vi "SerialServer.vi"(4 "STOP REF":refnum<vi>, 6 "Local Port":u16=16505, 7 "FPGA REF (DBDE)":T1) -> ()   [LabVIEW 2015]
uses:
  Controls (HOST)/FPGA REF (MWT).ctl
panel:
  out "Baud Rate":i32(ring)=1 items=["9600"=1, "19200"=2, "38400"=4, "57600"=8, "115200"=16, "230400"=32, "460800"=64, "921600"=128]
  out "error out":errorcluster
  out "OverRunError":bool
  in  "Flush on Close":bool
  out "UART TX count":u64
  out "UART RX count":u64
  out "TCP Bytes Out":u64
  out "Elements in UART TX Queue":i32
  out "Elements in UART RX Queue":i32
  out "TCP Bytes In":u64
  out "connection ID":refnum<k5>
  out "Connected?":bool
  out "Stopped?":bool caption="BeenStopped?"
  out "Remote Address":string
  out "Remote Port":u16
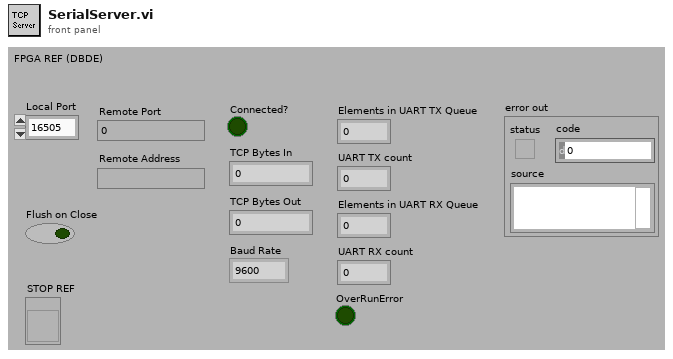
[diagram p1: front panel]
types:
  T1 = typedef "FPGA REF (MWT).ctl" = refnum<k20>
  T2 = enum16{"Standard", "Buffered", "CRLF", "Immediate"}
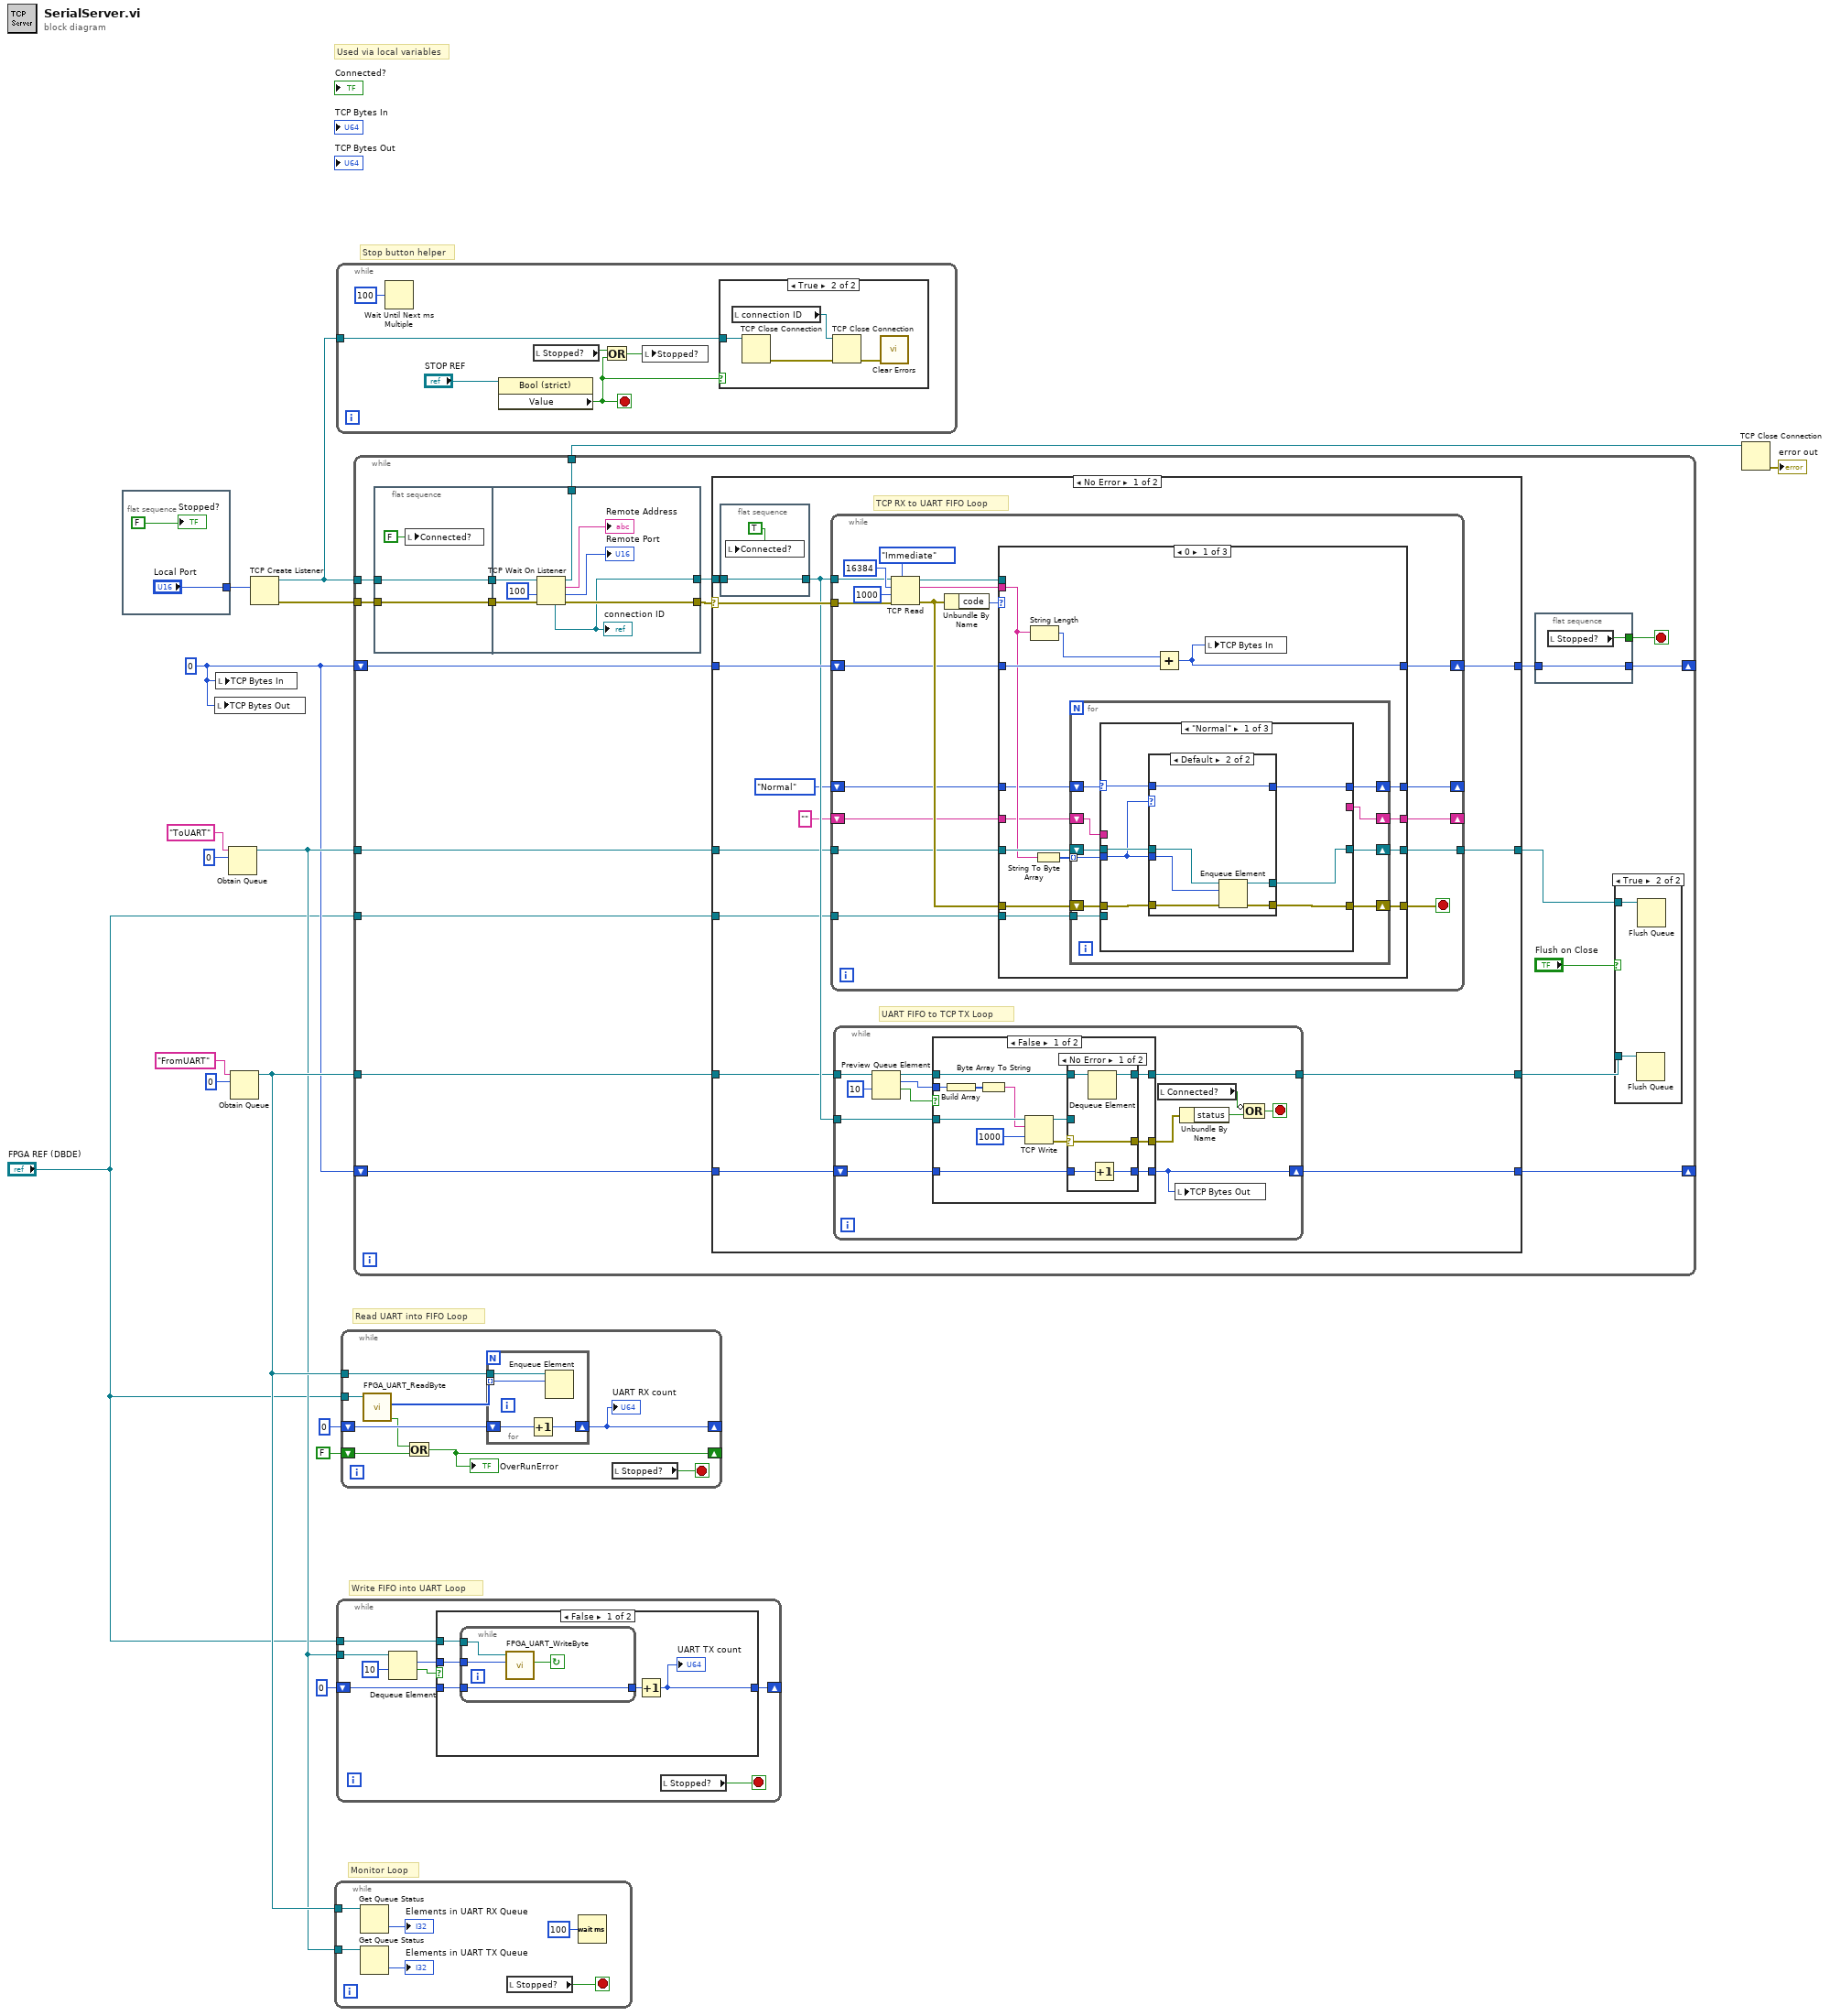
[diagram p0: block diagram]
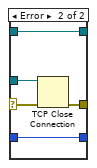
[diagram p5: hidden frame]
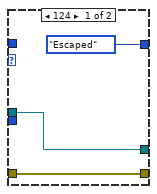
[diagram p7: hidden frame]
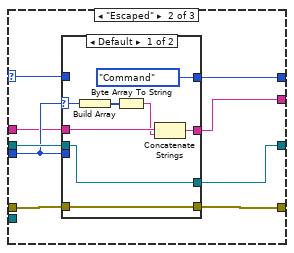
[diagram p8: hidden frame]
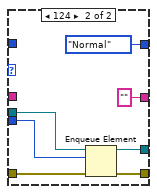
[diagram p9: hidden frame]
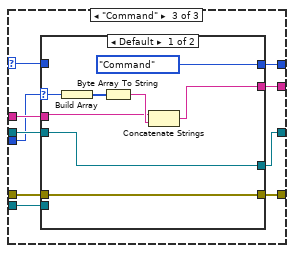
[diagram p10: hidden frame]
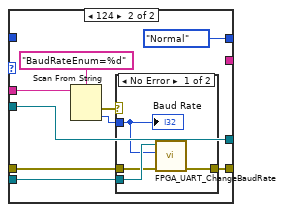
[diagram p11: hidden frame]
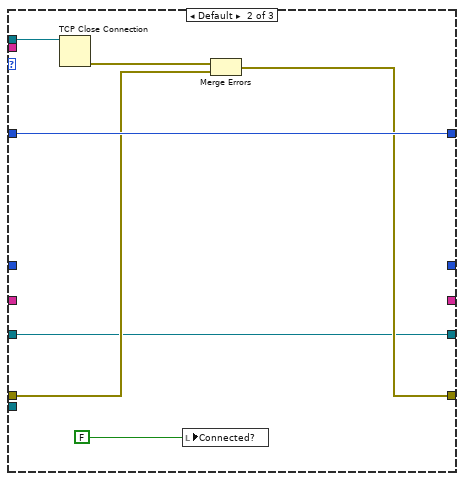
[diagram p13: hidden frame]
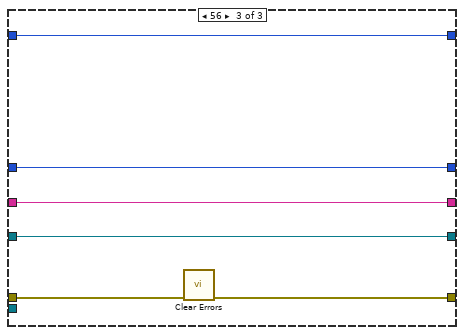
[diagram p14: hidden frame]
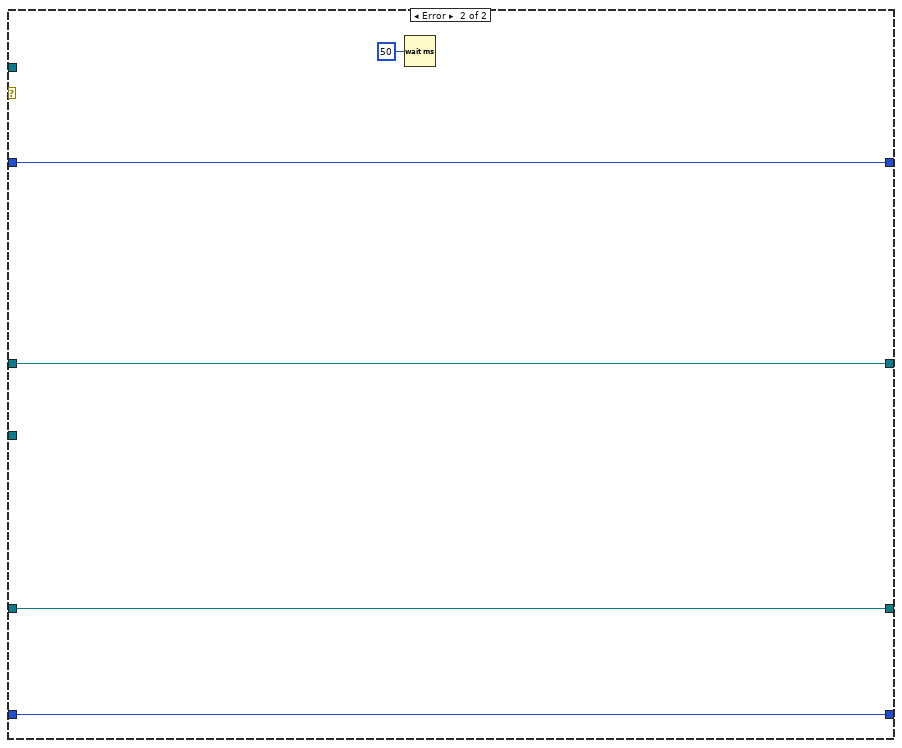
[diagram p15: hidden frame]
diagram:
  w8 = u64 0
  # "Monitor Loop"
  # "Write FIFO into UART Loop"
  # "Read UART into FIFO Loop"
  # "Stop button helper"
  # "Used via local variables"
  n1 = flat-sequence {
    tunnel: ["Local Port"] -> w3
    frame #0 {
      "Stopped?" <- FALSE ("Stopped?")
    }
  }
  n2 = local write "TCP Bytes Out"(w8) -> ()
  n3 = local write "TCP Bytes In"(w8) -> ()
  n4 = Obtain Queue(name (unnamed)="ToUART", element data type=u8 0) -> (queue out=w9:refnum<queue>)  [unwired: 3 in, 2 out]
  n5 = Obtain Queue(name (unnamed)="FromUART", element data type=u8 0) -> (queue out=w10:refnum<queue>)  [unwired: 3 in, 2 out]
  n6 = TCP Create Listener(10:w3) -> (0:w16:errorcluster, 3:w15:refnum<k5>)  [unwired: 1 in, 4 out]
  n7 = while {
    tunnel: w10 -> [w22]
    tunnel: w9 -> [w20]
    stop <- w24 stop-if-true
    n8 = Get Queue Status(queue=w22) -> (# elements in queue=→"Elements in UART RX Queue":i32)  [unwired: 1 in, 8 out]
    n9 = Get Queue Status(queue=w20) -> (# elements in queue=→"Elements in UART TX Queue":i32)  [unwired: 1 in, 8 out]
    n10 = local read "Stopped?"() -> (w24:bool)
    n11 = Wait (ms)(milliseconds to wait=u32 100) -> ()  [unwired: 1 out]
  }
  n12 = while {
    tunnel: w15 -> [w29]
    stop <- w26 stop-if-true
    n13 = Wait Until Next ms Multiple(millisecond multiple=u32 100) -> ()  [unwired: 1 out]
    n14 = property class="Bool (strict)"(reference="STOP REF") -> ("Value"=w26:bool)  [unwired: 1 in, 2 out]
    n15 = local read "Stopped?"() -> (w27:bool)
    n16 = Or(x=w27, y=w26) -> (x .or. y?=w28:bool)
    n17 = local write "Stopped?"(w28) -> ()
    n18 = case shown="True" w26 {
      tunnel: w29 -> [_ w31]
      frame False {
      }
      frame True {
        n19 = local read "connection ID"() -> (w33:refnum<k5>)
        n20 = TCP Close Connection(connection ID=w31) -> (error out=w32:errorcluster)  [unwired: 1 in, 2 out]
        n21 = TCP Close Connection(connection ID=w33, error in (no error)=w32) -> (error out=w34:errorcluster)  [unwired: 2 out]
        n22 = call <vilib>:"Clear Errors.vi"("error in (no error)"=w34) -> ()  [unwired: 1 in, 6 out]
      }
    }
  }
  n23 = while {
    tunnel: w9 -> [w42]
    shift-right: [w36] -> _
    shift-left: u64 0 -> [w37]
    tunnel: "FPGA REF (DBDE)" -> [w35]
    stop <- w38 stop-if-true
    n24 = Dequeue Element(queue=w42, timeout in ms (-1)=10) -> (element=w39:u8, timed out?=w40:bool)  [unwired: 1 in, 2 out]
    n25 = case shown="False" w40 {
      tunnel: w39 -> [w47 _]
      tunnel: w37 -> [w46 w52]
      tunnel: [w44 w52] -> w36
      tunnel: w35 -> [w43 _]
      frame False {
        n26 = while {
          tunnel: w47 -> [w50]
          tunnel: w46 -> [w51]
          tunnel: [w51] -> w45
          tunnel: w43 -> [w48]
          stop <- w49 continue-if-true
          n27 = call "FPGA_UART_WriteByte.vi"("Byte Value"=w50, "FPGA REF (DBDE)"=w48) -> ("Overflow?"=w49:bool)  [unwired: 1 in, 7 out]
        }
        n28 = Increment(x=w45) -> (x+1=w44:u64)
        "UART TX count" <- w44
      }
      frame True {
      }
    }
    n29 = local read "Stopped?"() -> (w38:bool)
  }
  n30 = while {
    tunnel: w10 -> [w60]
    shift-right: [w58] -> _
    shift-left: u64 0 -> [w59]
    tunnel: "FPGA REF (DBDE)" -> [w53]
    shift-right: [w54] -> _
    shift-left: FALSE -> [w55]
    stop <- w61 stop-if-true
    n31 = call "FPGA_UART_ReadByte.vi"("FPGA REF (DBDE)"=w53) -> ("OverRunError"=w56:bool, "Bytes"=w57:u8[])  [unwired: 9 out]
    n32 = Or(x=w56, y=w55) -> (x .or. y?=w54:bool)
    "OverRunError" <- w54
    n33 = for {
      tunnel: w60 -> [w65]
      tunnel: w57 -> [w62] mode=indexing
      shift-right: [w63] -> w58
      shift-left: w59 -> [w64]
      n34 = Increment(x=w64) -> (x+1=w63:u64)
      n35 = Enqueue Element(queue=w65, element=w62) -> ()  [unwired: 1 in, 4 out]
    }
    "UART RX count" <- w58
    n36 = local read "Stopped?"() -> (w61:bool)
  }
  n37 = while {
    tunnel: w15 -> [w83]
    tunnel: w16 -> [w84]
    shift-right: [w77] -> _
    shift-left: w8 -> [w79]
    tunnel: w9 -> [w76]
    tunnel: w10 -> [w73]
    shift-right: [w71] -> _
    shift-left: w8 -> [w72]
    tunnel: [w67] -> w5
    tunnel: "FPGA REF (DBDE)" -> [w66]
    stop <- w80 stop-if-true
    n38 = flat-sequence {
      tunnel: w83 -> [w88]
      tunnel: w84 -> [w89]
      tunnel: [w89] -> w75
      tunnel: [w88] -> w74
      tunnel: w75 -> [w95]
      tunnel: w74 -> [w94]
      tunnel: [w93] -> w82
      tunnel: [w90] -> w81
      tunnel: [w91] -> w67
      frame #0 {
        n39 = local write "Connected?"(FALSE ("Connected?")) -> ()
      }
      frame #1 {
        n40 = TCP Wait On Listener(8:w95, 9:100 ("timeout ms (wait forever: -1)"), 11:w94) -> (0:w93:errorcluster, 1:→"Remote Port":u16, 2:→"Remote Address":string, 3:w91:refnum<k5>, 4:w90:refnum<k5>)  [unwired: 1 in]
        "connection ID" <- w90
      }
    }
    n41 = case shown="No Error" w82 {
      selector: w82 -> [w111 _]
      tunnel: w81 -> [w110 _]
      tunnel: w79 -> [w113 w285]
      tunnel: [w112 w285] -> w78
      tunnel: w76 -> [w105 w282]
      tunnel: w73 -> [w106 w283]
      tunnel: w72 -> [w108 w284]
      tunnel: [w107 w284] -> w71
      tunnel: [w104 w282] -> w70
      tunnel: [w103 w283] -> w69
      tunnel: w66 -> [w101 _]
      frame No Error {
        # "UART FIFO to TCP TX Loop"
        # "TCP RX to UART FIFO Loop"
        n42 = flat-sequence {
          tunnel: w110 -> [w151]
          tunnel: [w151] -> w109
          frame #0 {
            n43 = local write "Connected?"(TRUE ("Connected?")) -> ()
          }
        }
        n44 = while {
          tunnel: w111 -> [w164]
          shift-right: [w161] -> w112
          shift-left: w113 -> [w162]
          tunnel: w105 -> [w160]
          tunnel: w109 -> [w159]
          tunnel: [w158] -> w104
          shift-right: [w153] -> _
          shift-left: "" -> [w157]
          shift-right: [w154] -> _
          shift-left: enum16{"Normal", "Escaped", "Command"}."Normal" -> [w156]
          tunnel: w101 -> [w155]
          stop <- w165 stop-if-true
          n45 = TCP Read(connection ID=w159, bytes to read=16384, error in (no error)=w164, 7:T2."Immediate" ("mode (standard)"), 9:1000 ("timeout ms (25000)")) -> (connection ID out=w167:refnum<k5>, data out=w166:string, error out=w168:errorcluster)
          n46 = Unbundle By Name(w168) -> ("code"=w169:i32)
          n47 = case shown="0" w169 {
            tunnel: w168 -> [w179 w272 w280]
            tunnel: w167 -> [_ w273 _]
            tunnel: w166 -> [w181 _ _]
            tunnel: [w178 w270 w279] -> w165
            tunnel: w162 -> [w185 w274 w278]
            tunnel: [w184 w274 w278] -> w161
            tunnel: w160 -> [w183 w268 w277]
            tunnel: [w177 w268 w277] -> w158
            tunnel: w157 -> [w176 _ w275]
            tunnel: w156 -> [w175 _ w276]
            tunnel: w155 -> [w174 _ _]
            tunnel: [w173 _ w276] -> w154
            tunnel: [w172 _ w275] -> w153
            frame 0 {
              n48 = String Length(string=w181) -> (length=w182:i32)
              n49 = String To Byte Array(string=w181) -> (unsigned byte array=w180:u8[])
              n50 = for {
                tunnel: w180 -> [w191] mode=indexing
                shift-right: [w193] -> w178
                shift-left: w179 -> [w194]
                shift-right: [w192] -> w177
                shift-left: w183 -> [w195]
                shift-right: [w186] -> w172
                shift-left: w176 -> [w188]
                shift-right: [w189] -> w173
                shift-left: w175 -> [w190]
                tunnel: w174 -> [w187]
                n51 = case shown="\"Normal\"" w190 {
                  selector: w190 -> [w196 w214 w240]
                  tunnel: w195 -> [w202 w220 w245]
                  tunnel: w191 -> [w198 w216 w237]
                  tunnel: w194 -> [w201 w219 w244]
                  tunnel: [w200 w218 w243] -> w193
                  tunnel: [w199 w217 w242] -> w192
                  tunnel: [w197 w215 w241] -> w189
                  tunnel: w188 -> [_ w213 w239]
                  tunnel: w187 -> [_ _ w238]
                  tunnel: [_ w212 w236] -> w186
                  frame "Normal" {
                    n52 = case shown="Default" w198 {
                      tunnel: w202 -> [w204 w211]
                      tunnel: w198 -> [_ w210]
                      tunnel: w201 -> [w203 w209]
                      tunnel: [w203 w208] -> w200
                      tunnel: [w204 w207] -> w199
                      tunnel: [enum16{"Normal", "Escaped", "Command"}."Escaped" w206] -> w197
                      tunnel: w196 -> [_ w206]
                      frame 124 {
                      }
                      frame Default {
                        n53 = Enqueue Element(queue=w211, element=w210, error in (no error)=w209) -> (queue out=w207:refnum<queue>, error out=w208:errorcluster)  [unwired: 2 out]
                      }
                    }
                  }
                  frame "Escaped" {
                    n54 = case shown="Default" w216 {
                      selector: w216 -> [w225 _]
                      tunnel: w220 -> [w227 w235]
                      tunnel: w216 -> [_ w234]
                      tunnel: w219 -> [w226 w233]
                      tunnel: [w226 w232] -> w218
                      tunnel: [w227 w231] -> w217
                      tunnel: [enum16{"Normal", "Escaped", "Command"}."Command" enum16{"Normal", "Escaped", "Command"}."Normal"] -> w215
                      tunnel: w214 -> [_ _]
                      tunnel: w213 -> [w223 _]
                      tunnel: [w221 ""] -> w212
                      frame Default {
                        n55 = Build Array(w225) -> (w224:u8[])
                        n56 = Byte Array To String(unsigned byte array=w224) -> (string=w222:string)
                        n57 = Concatenate Strings(w223, w222) -> (w221:string)
                      }
                      frame 124 {
                        n58 = Enqueue Element(queue=w235, element=w234, error in (no error)=w233) -> (queue out=w231:refnum<queue>, error out=w232:errorcluster)  [unwired: 2 out]
                      }
                    }
                  }
                  frame "Command" {
                    n59 = case shown="Default" w237 {
                      selector: w237 -> [w250 _]
                      tunnel: w245 -> [w252 w261]
                      tunnel: w244 -> [w251 w256]
                      tunnel: [w251 w255] -> w243
                      tunnel: [w252 w261] -> w242
                      tunnel: [enum16{"Normal", "Escaped", "Command"}."Command" enum16{"Normal", "Escaped", "Command"}."Normal"] -> w241
                      tunnel: w240 -> [_ _]
                      tunnel: w239 -> [w247 w254]
                      tunnel: w238 -> [_ w257]
                      tunnel: [w246 _] -> w236
                      frame Default {
                        n60 = Build Array(w250) -> (w249:u8[])
                        n61 = Byte Array To String(unsigned byte array=w249) -> (string=w248:string)
                        n62 = Concatenate Strings(w247, w248) -> (w246:string)
                      }
                      frame 124 {
                        n63 = Scan From String(format string="BaudRateEnum=%d", input string=w254) -> (error out=w259:errorcluster, output 1=w258:i32)  [unwired: 3 in, 2 out]
                        n64 = case shown="No Error" w259 {
                          tunnel: w258 -> [w263 _]
                          tunnel: w257 -> [w266 _]
                          tunnel: w256 -> [w265 w267]
                          tunnel: [w264 w267] -> w255
                          frame No Error {
                            n65 = call "FPGA_UART_ChangeBaudRate.vi"("error  in"=w265, "Baud Rate Enum"=w263, "FPGA VI Reference In"=w266) -> ("error out"=w264:errorcluster)  [unwired: 6 in, 1 out]
                            "Baud Rate" <- w263
                          }
                          frame Error {
                          }
                        }
                      }
                    }
                  }
                }
              }
              n66 = Add(x=w182, y=w185) -> (x+y=w184:u64)
              n67 = local write "TCP Bytes In"(w184) -> ()
            }
            frame Default {
              n68 = TCP Close Connection(connection ID=w273) -> (error out=w271:errorcluster)  [unwired: 1 in, 2 out]
              n69 = local write "Connected?"(FALSE ("Connected?")) -> ()
              n70 = Merge Errors(w271, w272) -> (w270:errorcluster)
            }
            frame 56 {
              n71 = call <vilib>:"Clear Errors.vi"("error in (no error)"=w280) -> ("error out"=w279:errorcluster)  [unwired: 1 in, 5 out]
            }
          }
        }
        n72 = while {
          tunnel: w109 -> [w122]
          tunnel: w106 -> [w125]
          tunnel: [w114] -> w103
          shift-right: [w118] -> w107
          shift-left: w108 -> [w120]
          stop <- w115 stop-if-true
          n73 = Preview Queue Element(queue=w125, timeout in ms (-1)=10) -> (queue out=w119:refnum<queue>, element=w123:u8, timed out?=w124:bool)  [unwired: 1 in, 1 out]
          n74 = case shown="False" w124 {
            tunnel: w123 -> [w137 _]
            tunnel: w122 -> [w138 _]
            tunnel: [w132 _] -> w121
            tunnel: w120 -> [w129 w150]
            tunnel: [w128 w150] -> w118
            tunnel: w119 -> [w130 w149]
            tunnel: [w127 w149] -> w114
            frame False {
              n75 = Build Array(w137) -> (w136:u8[])
              n76 = Byte Array To String(unsigned byte array=w136) -> (string=w135:string)
              n77 = TCP Write(connection ID=w138, data in=w135, 9:1000 ("timeout ms (25000)")) -> (connection ID out=w131:refnum<k5>, error out=w133:errorcluster)  [unwired: 1 in, 1 out]
              n78 = case shown="No Error" w133 {
                selector: w133 -> [w143 w147]
                tunnel: [w143 w146] -> w132
                tunnel: w131 -> [_ w148]
                tunnel: w130 -> [w142 w144]
                tunnel: w129 -> [w141 w145]
                tunnel: [w140 w145] -> w128
                tunnel: [w139 w144] -> w127
                frame No Error {
                  n79 = Dequeue Element(queue=w142) -> (queue out=w139:refnum<queue>)  [unwired: 2 in, 3 out]
                  n80 = Increment(x=w141) -> (x+1=w140:u64)
                }
                frame Error {
                  n81 = TCP Close Connection(connection ID=w148, error in (no error)=w147) -> (error out=w146:errorcluster)  [unwired: 2 out]
                }
              }
            }
            frame True {
            }
          }
          n82 = local read "Connected?"() -> (w117:bool)
          n83 = local write "TCP Bytes Out"(w118) -> ()
          n84 = Unbundle By Name(w121) -> ("status"=w116:bool)
          n85 = Compound Arithmetic op=OR(invert w117, w116) -> (w115:bool)
        }
      }
      frame Error {
        n86 = Wait (ms)(milliseconds to wait=u32 50) -> ()  [unwired: 1 out]
      }
    }
    n87 = flat-sequence {
      tunnel: [w99] -> w80
      tunnel: w78 -> [w98]
      tunnel: [w98] -> w77
      frame #0 {
        n88 = local read "Stopped?"() -> (w99:bool)
      }
    }
    n89 = case shown="True" "Flush on Close" {
      tunnel: w70 -> [_ w86]
      tunnel: w69 -> [_ w85]
      frame False {
      }
      frame True {
        n90 = Flush Queue(queue=w85) -> ()  [unwired: 1 in, 3 out]
        n91 = Flush Queue(queue=w86) -> ()  [unwired: 1 in, 3 out]
      }
    }
  }
  n92 = TCP Close Connection(connection ID=w5) -> (error out=→"error out":errorcluster)  [unwired: 2 in, 1 out]
